vi "Caller.vi"(5 "Initialize-Error Passback":refnum<notifier>, 7 "Events Passback":refnum<notifier>, 8 "Caller":T1, 9 "Did Stop Enqueuer":refnum<user-event>, 10 "Launch":refnum<notifier>, 11 "Actor in":refnum<class "Actor.lvclass">) -> ()   [LabVIEW 2018, in "Scripting.lvlib" / "Actor.lvclass"]
uses:
  Actor.lvclass
  Message-Enqueuer References.ctl
  Stop.ctl
  Launch.ctl
  Did Initialize.ctl
  Did Stop.ctl
  Front-Panel State.ctl
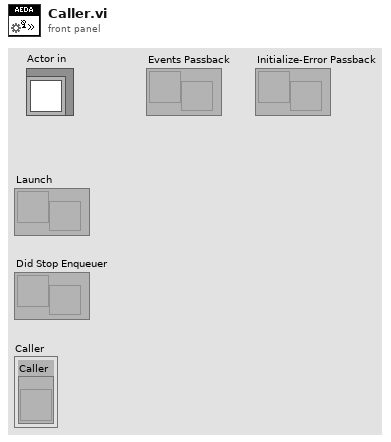
[diagram p1: front panel]
types:
  T1 = typedef "Scripting.lvlib/Actor.lvclass/Launch.ctl" = cluster{"Caller":refnum<vi>}
  T2 = typedef "Scripting.lvlib/Actor.lvclass/Did Stop.ctl" = cluster{"State":refnum<class "Actor.lvclass">, "Final Error":errorcluster}
  T3 = typedef "Scripting.lvlib/Actor.lvclass/Messages.ctl" = refnum<event-registration>
  T4 = typedef "Scripting.lvlib/Actor.lvclass/Message-Enqueuer References.ctl" = cluster{"Stop":refnum<user-event>, "Launch":refnum<user-event>, "Did Initialize":refnum<user-event>}
  T5 = typedef "Scripting.lvlib/Actor.lvclass/Front-Panel State.ctl" = enum16{"Don't Show", "Show"}
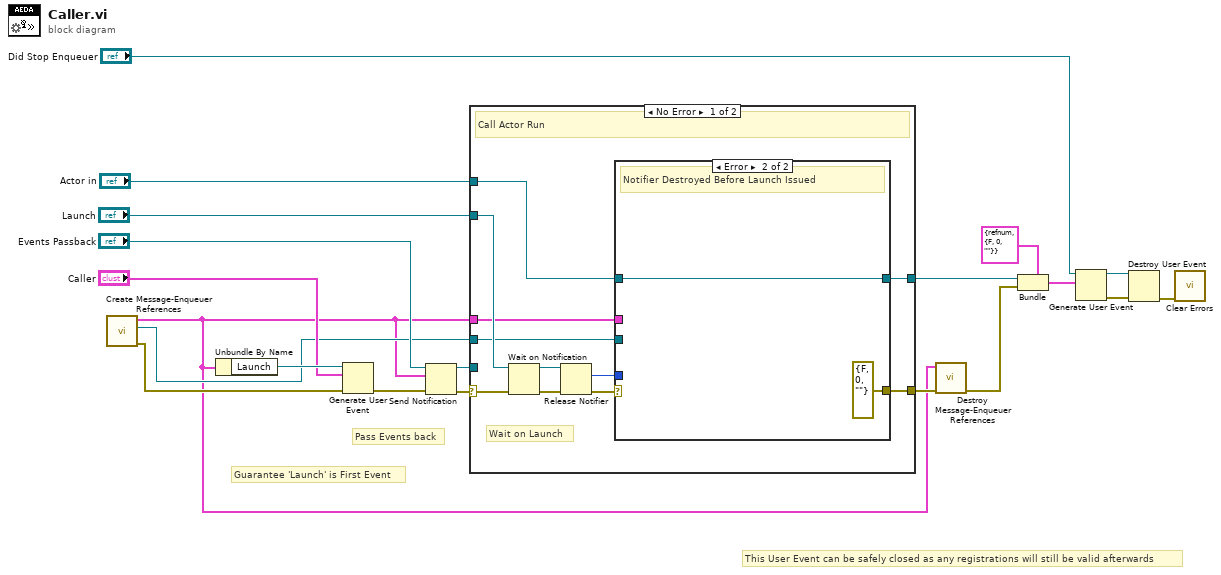
[diagram p0: block diagram]
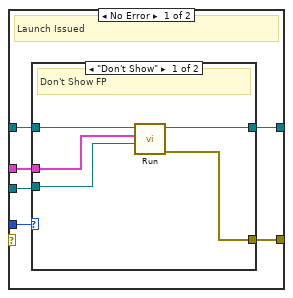
[diagram p2: hidden frame]
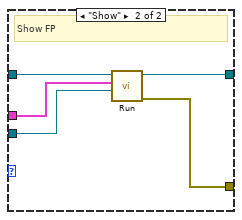
[diagram p3: hidden frame]
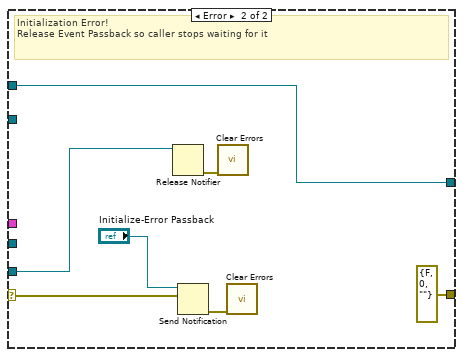
[diagram p4: hidden frame]
diagram:
  # "This User Event can be safely closed as any registrations will still be valid afterwards"
  # "Guarantee 'Launch' is First Event"
  # "Pass Events back"
  n1 = call "Create Message-Enqueuer References.vi"() -> ("error out"=w10:errorcluster, "Messages"=w11:T3, "API"=w4:T4)  [unwired: 9 in]
  n2 = Unbundle By Name(w4) -> ("Launch"=w16:refnum<user-event>)
  n3 = Generate User Event(user event=w16, event data cluster="Caller", error in=w10) -> (error out=w15:errorcluster)  [unwired: 1 in, 1 out]
  n4 = Send Notification(notification=w4, notifier="Events Passback", error in (no error)=w15) -> (notifier out=w7:refnum<notifier>, error out=w14:errorcluster)
  n5 = case shown="No Error" w14 {
    selector: w14 -> [w29 w52]
    tunnel: "Launch" -> [w31 _]
    tunnel: "Actor in" -> [w30 w56]
    tunnel: w4 -> [w28 _]
    tunnel: w11 -> [w27 _]
    tunnel: [w21 errorcluster {"status"=FALSE, "code"=0, "source"=""} ("error out")] -> w6
    tunnel: [w26 w56] -> w8
    tunnel: w7 -> [_ w55]
    frame No Error {
      # "Wait on Launch"
      # "Call Actor Run"
      n6 = Wait on Notification(notifier=w31, error in (no error)=w29) -> (notifier out=w24:refnum<notifier>, error out=w25:errorcluster)  [unwired: 2 in, 2 out]
      n7 = Release Notifier(notifier=w24, error in (no error)=w25) -> (last notification=w23:T5, error out=w22:errorcluster)  [unwired: 1 in, 1 out]
      n8 = case shown="Error" w22 {
        tunnel: w30 -> [w37 w49]
        tunnel: [w36 w49] -> w26
        tunnel: [w35 errorcluster {"status"=FALSE, "code"=0, "source"=""} ("error out")] -> w21
        tunnel: w28 -> [w34 _]
        tunnel: w27 -> [w33 _]
        tunnel: w23 -> [w32 _]
        frame No Error {
          # "Launch Issued"
          n9 = case shown="\"Don't Show\"" w32 {
            tunnel: w37 -> [w42 w47]
            tunnel: [w41 w45] -> w35
            tunnel: [w40 w46] -> w36
            tunnel: w34 -> [w39 w44]
            tunnel: w33 -> [w38 w43]
            frame "Don't Show" {
              # "Don't Show FP"
              n10 = call-dynamic "Run.vi"("Messages"=w38, "Message-Enqueue Refs"=w39, "Actor in"=w42) -> ("error out"=w41:errorcluster, "Actor out"=w40:refnum<class "Actor.lvclass">)  [unwired: 7 in]
            }
            frame "Show" {
              # "Show FP"
              n11 = call-dynamic "Run.vi"("Messages"=w43, "Message-Enqueue Refs"=w44, "Actor in"=w47) -> ("error out"=w45:errorcluster, "Actor out"=w46:refnum<class "Actor.lvclass">)  [unwired: 7 in]
            }
          }
        }
        frame Error {
          # "Notifier Destroyed Before Launch Issued"
        }
      }
    }
    frame Error {
      # "Initialization Error!\nRelease Event Passback so caller stops waiting for it"
      n12 = Release Notifier(notifier=w55) -> (error out=w54:errorcluster)  [unwired: 2 in, 2 out]
      n13 = Send Notification(notification=w52, notifier="Initialize-Error Passback") -> (error out=w51:errorcluster)  [unwired: 1 in, 1 out]
      n14 = call <vilib>:"Clear Errors.vi"("error in (no error)"=w54) -> ()  [unwired: 5 in, 2 out]
      n15 = call <vilib>:"Clear Errors.vi"("error in (no error)"=w51) -> ()  [unwired: 5 in, 2 out]
    }
  }
  n16 = call "Destroy Message-Enqueuer References.vi"("error in (no error)"=w6, "Event-References"=w4) -> ("error out"=w5:errorcluster)  [unwired: 9 in]
  n17 = Bundle(cluster=T2 {"State"=refnum, "Final Error"={"status"=FALSE, "code"=0, "source"=""}} ("event data"), "State"=w8, "Final Error"=w5) -> (w20:T2)
  n18 = Generate User Event(user event="Did Stop Enqueuer", event data cluster=w20) -> (user event out=w3:refnum<user-event>, error out=w2:errorcluster)  [unwired: 2 in]
  n19 = Destroy User Event(user event=w3, error in=w2) -> (error out=w1:errorcluster)
  n20 = call <vilib>:"Clear Errors.vi"("error in (no error)"=w1) -> ()  [unwired: 5 in, 2 out]
